vi "Publish.vi"(8 "error in (no error)":errorcluster, 10 "Publish Group Data":T1, 11 "Telemetry Server in":refnum<class "Telemetry Server.lvclass">) -> (0 "error out":errorcluster, 3 "Telemetry Server out":refnum<class "Telemetry Server.lvclass">)   [LabVIEW 2020, in "VolatusTelemetry.lvlib" / "Telemetry Server.lvclass"]
uses:
  Telemetry Server.lvclass
  Telemetry Server.lvclass/Telemetry Server.ctl
  messages/UdpPayload/Data.ctl
  messages/UdpPayload/UdpPayload.lvlib
  VolatusTelemetry.lvlib
  lv-protoc/LV-Proto/Message/Message.lvclass
  lv-vecto/Vecto/Vecto.lvlib
  VolatusConfig/Group Type.ctl
  VolatusConfig/VolatusConfig.lvlib
  Publish Group Data.ctl
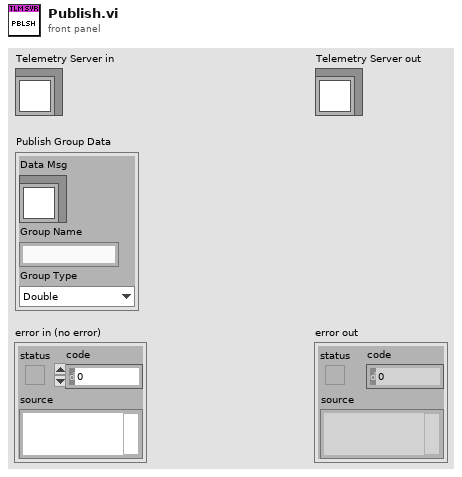
[diagram p1: front panel]
types:
  T1 = typedef "VolatusTelemetry.lvlib/Publish Group Data.ctl" = cluster{"Data Msg":refnum<class "Message.lvclass">, "Group Name":string, "Group Type":T2}
  T2 = typedef "VolatusConfig.lvlib/Group Type.ctl" = enum16{"Double", "Bool", "String"}
  T3 = typedef "UdpPayload.lvlib/Data.ctl" = cluster{"source_id":u32, "sequence":u32, "timestamp":i64, "type":string, "payload":u8[]}
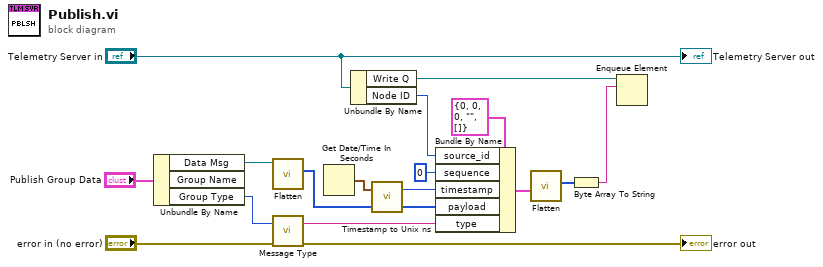
[diagram p0: block diagram]
diagram:
  n1 = Unbundle By Name("Publish Group Data") -> ("Data Msg"=w9:refnum<class "Message.lvclass">, "Group Type"=w10:T2)  [unwired: 1 out]
  n2 = call-dynamic "Flatten.vi"("Message in"=w9) -> ("Buffer"=w8:u8[])  [unwired: 8 in, 2 out]
  n3 = call "Message Type.vi"("Group Type"=w10) -> ("type"=w11:string)  [unwired: 6 in]
  n4 = Get Date/Time In Seconds() -> (seconds since 1Jan1904=w1:timestamp)
  n5 = Unbundle By Name("Telemetry Server in") -> ("Write Q"=w14:refnum<queue>, "Node ID"=w4:u32)
  n6 = call "Timestamp to Unix ns.vi"("Time Stamp"=w1) -> ("unix ns"=w2:i64)  [unwired: 2 in]
  n7 = Bundle By Name(cluster=T3 {"source_id"=0, "sequence"=0, "timestamp"=0, "type"="", "payload"=[]} ("UdpPayload"), "source_id"=w4, "sequence"=u32 0, "timestamp"=w2, "payload"=w8, "type"=w11) -> (w7:T3)
  n8 = call "Flatten.vi"("Data"=w7) -> ("Buffer"=w6:u8[])  [unwired: 9 in, 1 out]
  n9 = Byte Array To String(unsigned byte array=w6) -> (string=w5:string)
  n10 = Enqueue Element(queue=w14, element=w5) -> ()  [unwired: 2 in, 3 out]
  "error out" <- "error in (no error)"
  "Telemetry Server out" <- "Telemetry Server in"
